vi "EMV T7 Flow Detect 1.vi"(6 "Detect Flow Start?":bool, 7 "Detection Slope":dbl=0.2 format="%#_13g", 8 "error in (no error)":errorcluster, 9 "T7_DELTA_FLOW_THRESHOLD":dbl, 11 "Current T7 Temperatures":dbl[](array[numeric])) -> (0 "error out":errorcluster, 1 "slope":dbl, 2 "Detection?":bool, 3 "Current T7 Temperatures Output":dbl[](array[numeric]))   [LabVIEW 2016]
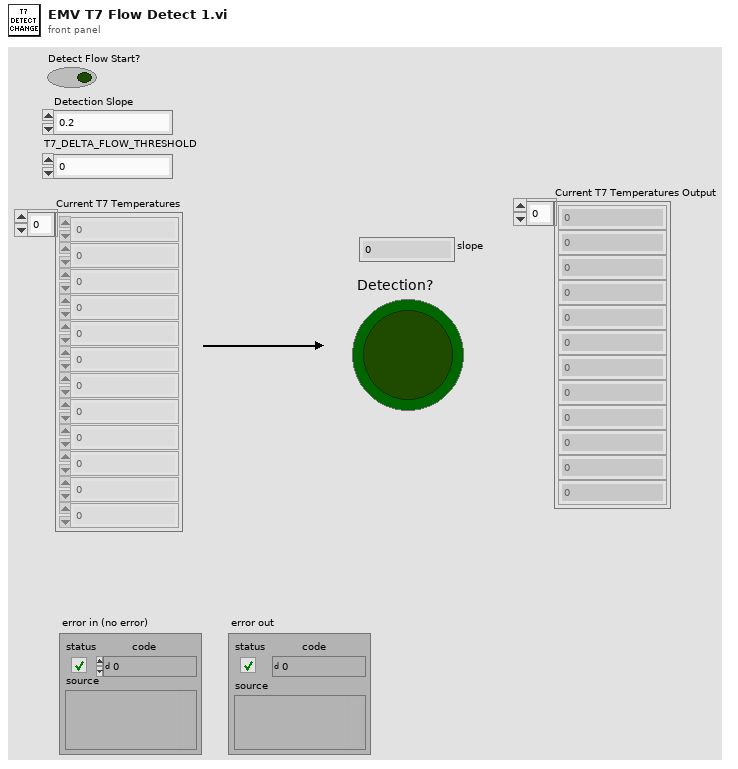
[diagram p1: front panel]
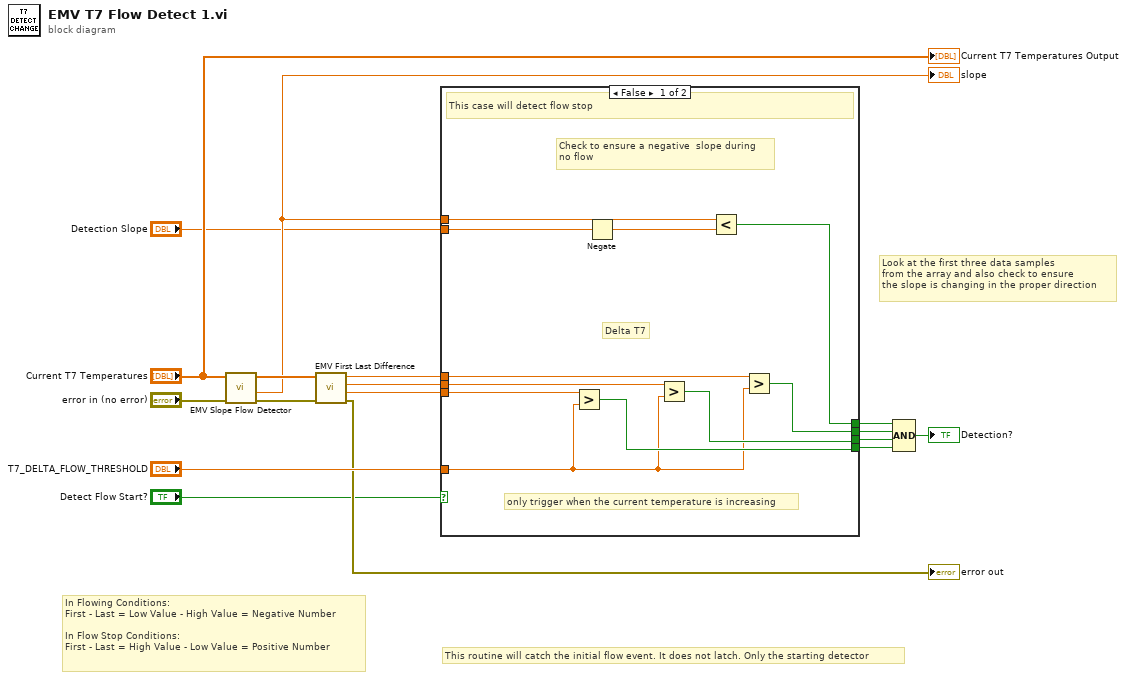
[diagram p0: block diagram]
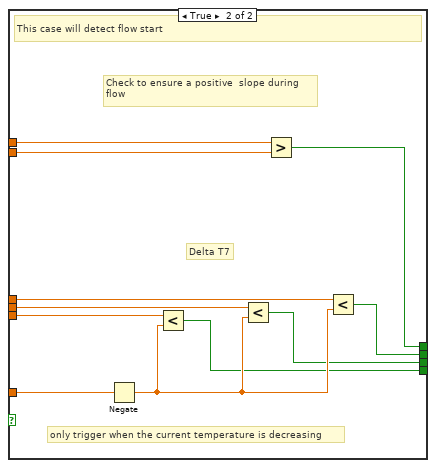
[diagram p2: hidden frame]
diagram:
  # "Look at the first three data samples \nfrom the array and also check to ensure\nthe slope is changing in the proper direction"
  # "In Flowing Conditions:\nFirst - Last = Low Value - High Value = Negative Number\n\nIn Flow Stop Conditions:\nFirst - Last = High Value - Low Value = Positive Number"
  # "This routine will catch the initial flow event. It does not latch. Only the starting detector"
  n1 = call "EMV Slope Flow Detector.vi"("error in (no error)"="error in (no error)", "Current T6 Temperatures in"="Current T7 Temperatures") -> ("error out"=w8:errorcluster, "slope"=w5:dbl, "Current T6 Temperatures out"=w7:dbl[])  [unwired: 7 in]
  "slope" <- w5
  n2 = call "EMV First Last Difference.vi"("error in (no error)"=w8, "Current T6 Temperatures in"=w7) -> ("error out"=→"error out":errorcluster, "First - Row 8"=w15:dbl, "First - Row 9"=w16:dbl, "First - Row 10"=w17:dbl)  [unwired: 5 in, 1 out]
  n3 = case shown="False" "Detect Flow Start?" {
    tunnel: w17 -> [w25 w39]
    tunnel: w16 -> [w26 w38]
    tunnel: w15 -> [w27 w37]
    tunnel: [w23 w35] -> w14
    tunnel: [w22 w34] -> w13
    tunnel: [w21 w33] -> w12
    tunnel: "T7_DELTA_FLOW_THRESHOLD" -> [w20 w32]
    tunnel: [w24 w31] -> w9
    tunnel: w5 -> [w28 w30]
    tunnel: "Detection Slope" -> [w19 w29]
    frame False {
      # "only trigger when the current temperature is increasing"
      # "Delta T7"
      # "Check to ensure a negative  slope during\nno flow"
      # "This case will detect flow stop"
      n4 = Greater?(x=w27, y=w20) -> (0:w21:bool)
      n5 = Negate(x=w19) -> (-x=w18:dbl)
      n6 = Greater?(x=w26, y=w20) -> (0:w22:bool)
      n7 = Less?(x=w28, y=w18) -> (x < y?=w24:bool)
      n8 = Greater?(x=w25, y=w20) -> (0:w23:bool)
    }
    frame True {
      # "Check to ensure a positive  slope during\nflow"
      # "only trigger when the current temperature is decreasing"
      # "Delta T7"
      # "This case will detect flow start"
      n9 = Negate(x=w32) -> (-x=w36:dbl)
      n10 = Less?(x=w37, y=w36) -> (x < y?=w33:bool)
      n11 = Less?(x=w38, y=w36) -> (x < y?=w34:bool)
      n12 = Greater?(x=w30, y=w29) -> (0:w31:bool)
      n13 = Less?(x=w39, y=w36) -> (x < y?=w35:bool)
    }
  }
  n14 = Compound Arithmetic op=AND(w9, w14, w13, w12) -> (→"Detection?":bool)
  "Current T7 Temperatures Output" <- "Current T7 Temperatures"
